vi "Scripting Set BD Color.vi"(8 "error in":errorcluster, 11 "Path":path) -> (0 "error out":errorcluster)   [LabVIEW 2026]
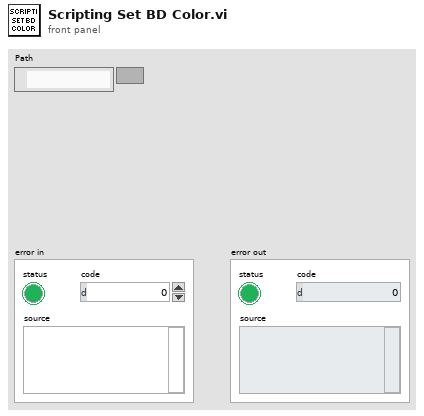
[diagram p1: front panel]
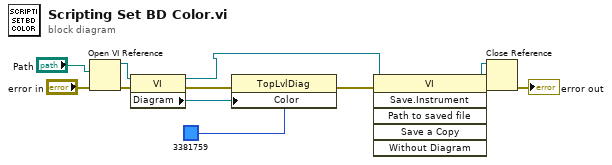
[diagram p0: block diagram]
diagram:
  n1 = Open VI Reference(vi path="Path", error in (no error)="error in") -> (vi reference=w5:refnum<vi>, error out=w11:errorcluster)  [unwired: 4 in]
  n2 = property class="VI"(reference=w5, error in=w11) -> (reference out=w2:refnum<vi>, error out=w6:errorcluster, "Diagram"=w3:refnum<vi>)
  n3 = property class="TopLvlDiag"(reference=w3, error in=w6, "Color"=u32 3381759) -> (error out=w4:errorcluster)  [unwired: 1 out]
  n4 = invoke class="VI" method="Save.Instrument"(reference=w2, error in=w4) -> (reference out=w7:refnum<vi>, error out=w10:errorcluster)  [unwired: 4 in, 4 out]
  n5 = Close Reference(reference=w7, error in (no error)=w10) -> (error out=→"error out":errorcluster)
